vi "Get Reserved Names.vi"() -> (2 "reserved names":string[](array[string])=["MeasurementService Editor", "MeasurementLink Measurement Template", "MeasurementLink Discovery Client", "MeasurementLink Measurement Server", "MeasurementLink Measurement Server Internal", "MeasurementLink Pin Map Client", "MeasurementLink Session Management Client", "grpc-lvsupport-release", "gRPC-servicer-release", "gRPC Template Creation Utility-release", "Client Template", "Service Template"])   [LabVIEW 2021, in "MeasurementService Editor.lvlib"]
uses:
  MeasurementService Editor.lvlib
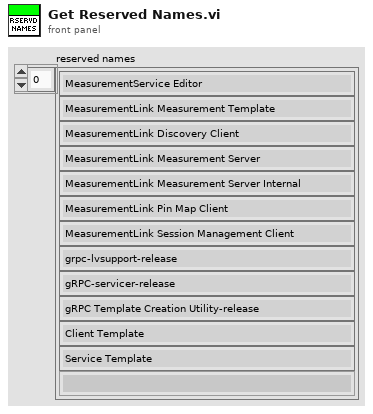
[diagram p1: front panel]
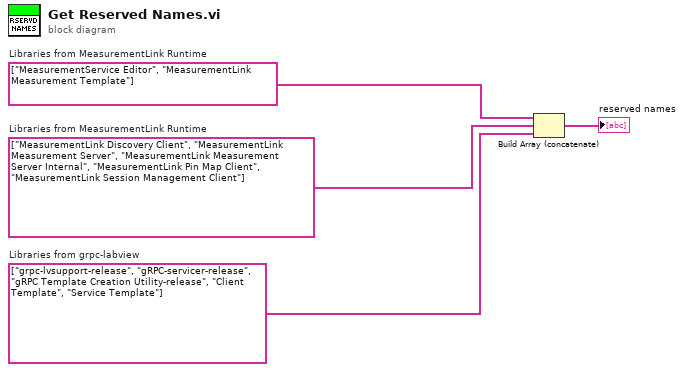
[diagram p0: block diagram]
diagram:
  w2 = string[] ["MeasurementService Editor", "MeasurementLink Measurement Template"]  # Libraries from MeasurementLink Runtime
  w4 = string[] ["grpc-lvsupport-release", "gRPC-servicer-release", "gRPC Template Creation Utility-release", "Client Template", "Service Template"]  # Libraries from grpc-labview
  w3 = string[] ["MeasurementLink Discovery Client", "MeasurementLink Measurement Server", "MeasurementLink Measurement Server Internal", "MeasurementLink Pin Map Client", "MeasurementLink Session Management Client"]  # Libraries from MeasurementLink Runtime
  n1 = Build Array (concatenate)(w2, w3, w4) -> (→"reserved names":string[])
